vi "LvIRKit_SUB_DataToString.vi"() -> ()   [LabVIEW 2014]
panel:
  out "Data[] out":T1(array[cluster])
  out "string":string
  in  "Data[]":T1(array[cluster])=[{"id"=1, "name"="ボタン1", "ircode"="{\"abc\":123}"}, {"id"=2, "name"="ボタン2", "ircode"="{\"abc\":456}"}]
  # "id は追加時に自動的に +1される。\nnameだけだとボタン名が重複する可能性があるから。\nデータが削除されると、空き番号になる。id は I32。そこまで数が登録されないと思う。"
  # "データの保存は、JSON文字列をテキスト保存する\n配列データだが、LabVIEW拡張を有効にして保存する。\n他のソフトからは利用できない。\n本当はSQLiteにしたかったが、SQLiteツールキットがJKIになっていて、\n開発環境にJKIが入ってなかったから、面倒なので使わないことにした。\n\nリモコンのコードも JSONだが特に加工しないでそのまま保存、そのまま送信する"
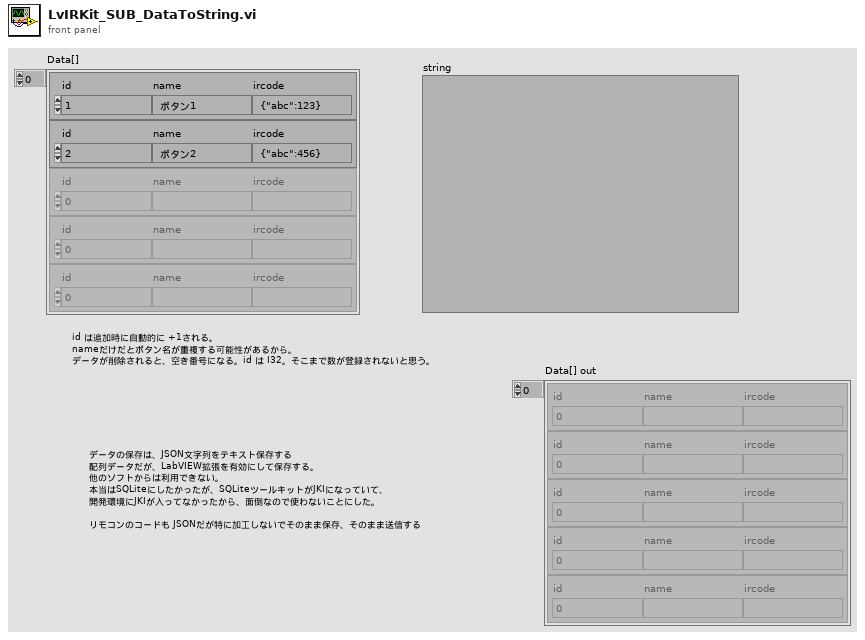
[diagram p1: front panel]
types:
  T1 = cluster{"id":i32, "name":string, "ircode":string}[]
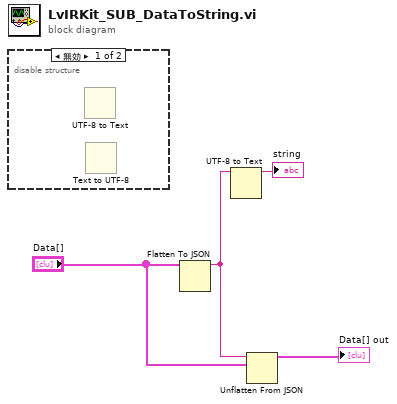
[diagram p0: block diagram]
diagram:
  n1 = disable-structure shown="無効" {
    frame Disabled {
      n2 = UTF-8 to Text() -> ()  [unwired: 3 in, 2 out]
      n3 = Text to UTF-8() -> ()  [unwired: 3 in, 2 out]
    }
    frame Enabled {
    }
  }
  n4 = Flatten To JSON(anything="Data[]") -> (JSON string=w2:string)  [unwired: 2 in, 1 out]
  n5 = UTF-8 to Text(11:w2) -> (3:→"string":string)  [unwired: 2 in, 1 out]
  n6 = Unflatten From JSON(JSON string=w2, type and defaults="Data[]") -> (value=→"Data[] out":T1)  [unwired: 5 in, 1 out]
